vi "SDG60ConfArbWaveform3.vi"(0 "VISA resource name":refnum<visa-resource-name>="USB0::0xF4EC::0x1101::SDG6XEBC5R0119::INSTR", 1 "DDS/TArb 0: DDS":i32(ring) items=["DDS", "TrueArb"], 2 "Interpolation 0: Zero-order":i32(ring) items=["Zero-Order", "Linear", "Sinc", "Sin27", "Sinc13"], 3 "Offset (0.00 V)":dbl min=-10.0 max=10.0 format="%#_15g", 5 "Select Channel (1:Channel 1)":i32(ring)=1 items=["Channel 1"=1, "Channel 2"=2], 7 "Amplitude(0.1 Vpp)":dbl=0.1 min=0.001 max=20.0 step=1.0 format="%#.15f", 9 "Freq/SR/P (1 Hz)":dbl=1.0 min=1e-06 max=160000000.0 step=1.0 format="%#.15g", 11 "error in (no error)":errorcluster, 12 "Select Freq/SR/P (0:Freq)":i32(ring) items=["Frequency", "Sample Rate", "Period"], 13 "Phase (0 deg)":dbl min=-360.0 max=360.0 format="%#.15g") -> (4 "VISA resource name out":refnum<visa-resource-name>, 15 "error out":errorcluster)   [LabVIEW 2018]
doc: "Sets the waveform parameters for an arbitrary waveform. This VI should be called after <b>Create Arbitrary Waveform.vi</b> (for user defined arbitrary waveform) and <b>Select Arbitrary Waveform.vi</b>"
panel:
  # "Must precede with SDG60SelectArbitraryWFM\nMay take time (~20s) if WFM is large"
  # "Sinc type interpolations use virtual keys\nVirtual keys not used for zero-hold & linear\nInterpolation method, is only for TrueArb\nIf still selected, generator will not make any parameter changes"
  # "Range: 2mVpp-20Vpp. \n6 digits precision"
  # "Range: -10V-10V\n6 digits precision"
  # "Freq (DDS): 1uHz-50MHz \nFreq (TrueArb): 1uHz- Max depends on WFM length\nSR: 1uS/s-300MSa/s\nP: 20ns-1Ms\n10 Digit precision for F & SR\n6 Digit precision for P"
  # "May need more testing, as had issues\nwhere some of the parameters didn't go\nthrough the first time round"
  # "For TrueArb use only F or SR \nFor DDS use F or P\nMay take time (seconds to tens of secons!) to switch to TrueArb if WFM is large"
  # "Range -360..360deg, larger values will be warped to this range. Resolution 0.0001 deg"
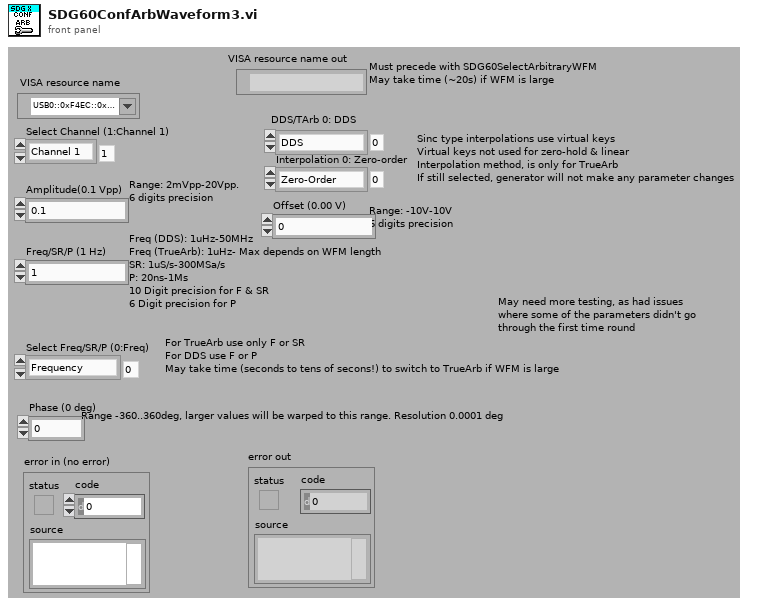
[diagram p1: front panel]
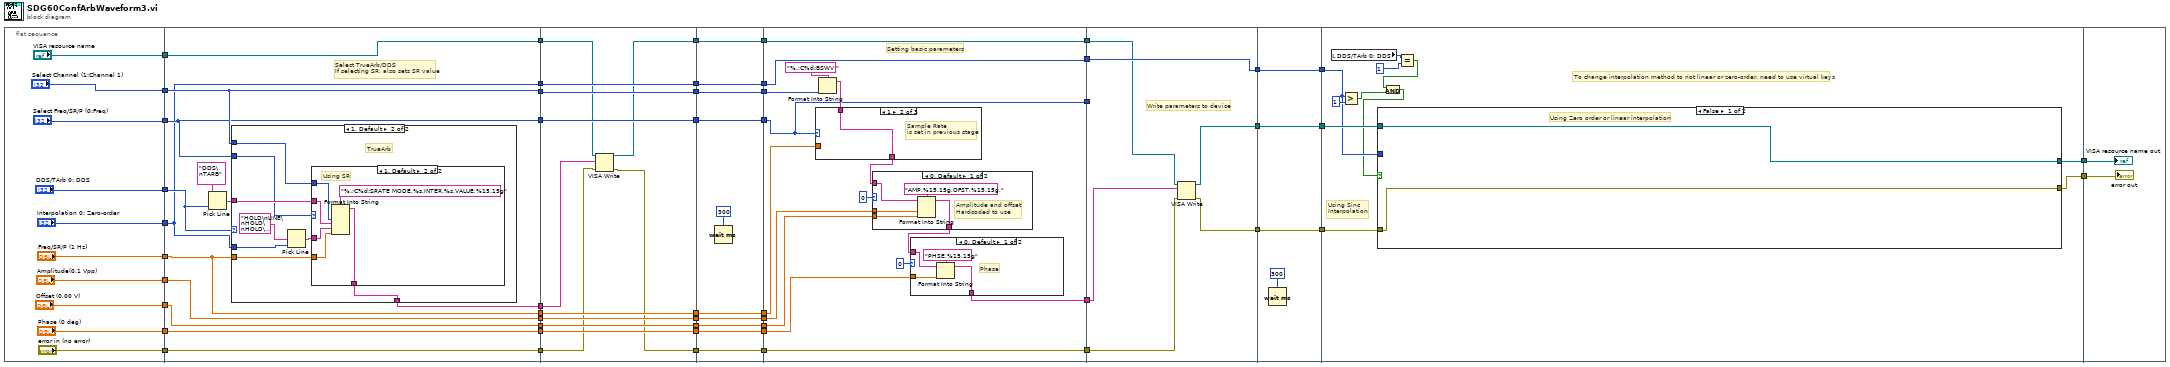
[diagram p0: block diagram]
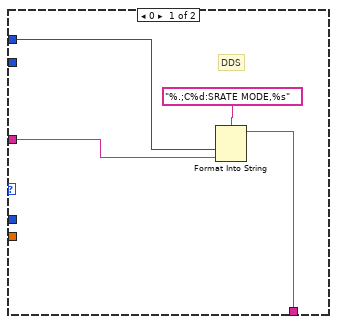
[diagram p2: hidden frame]
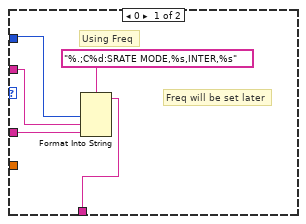
[diagram p3: hidden frame]
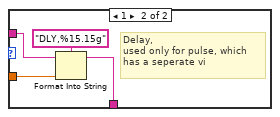
[diagram p4: hidden frame]
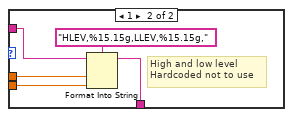
[diagram p5: hidden frame]
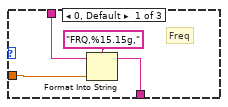
[diagram p6: hidden frame]
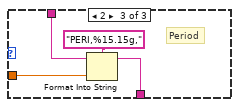
[diagram p7: hidden frame]
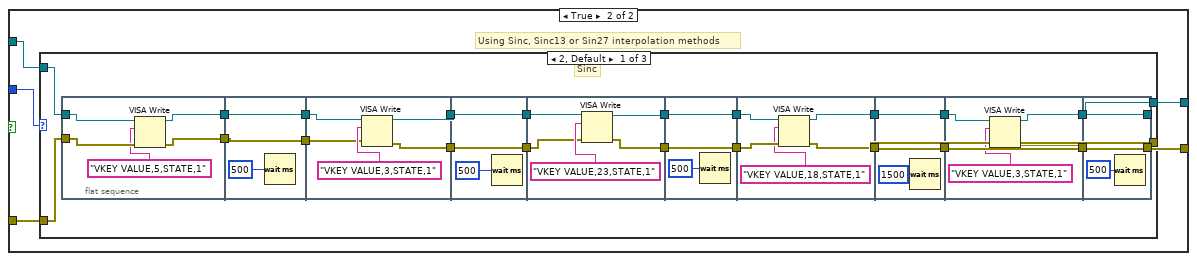
[diagram p8: hidden frame]
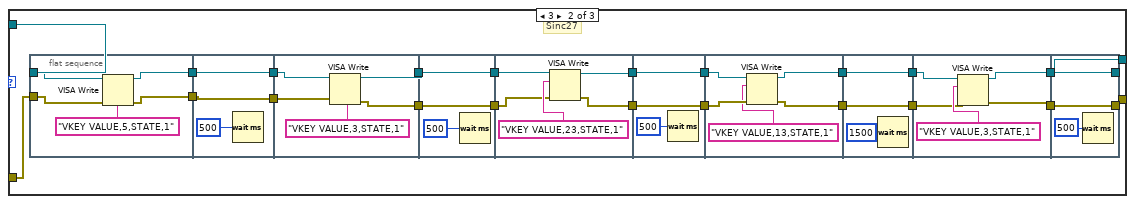
[diagram p9: hidden frame]
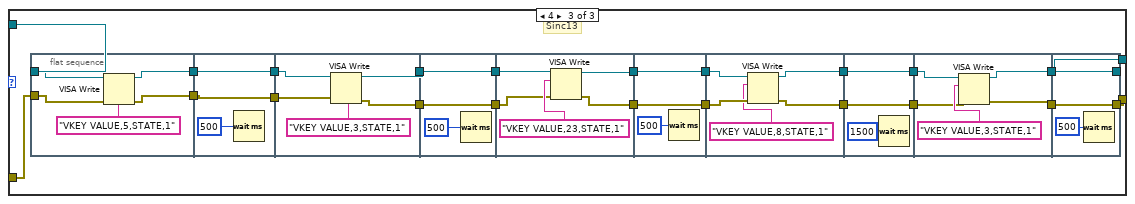
[diagram p10: hidden frame]
diagram:
  n1 = flat-sequence {
    tunnel: ["VISA resource name"] -> w51
    tunnel: ["error in (no error)"] -> w50
    tunnel: ["Amplitude(0.1 Vpp)"] -> w49
    tunnel: ["Phase (0 deg)"] -> w48
    tunnel: ["Freq/SR/P (1 Hz)"] -> w47
    tunnel: ["Offset (0.00 V)"] -> w46
    tunnel: ["Select Freq/SR/P (0:Freq)"] -> w45
    tunnel: ["DDS/TArb 0: DDS"] -> w44
    tunnel: ["Interpolation 0: Zero-order"] -> w43
    tunnel: ["Select Channel (1:Channel 1)"] -> w42
    tunnel: w51 -> [w70]
    tunnel: w50 -> [w74]
    tunnel: w49 -> [w68]
    tunnel: w48 -> [w69]
    tunnel: w47 -> [w67]
    tunnel: w46 -> [w66]
    tunnel: w45 -> [w64]
    tunnel: w44 -> [w71]
    tunnel: w43 -> [w63]
    tunnel: w42 -> [w65]
    tunnel: [w74] -> w34
    tunnel: [w70] -> w33
    tunnel: [w69] -> w32
    tunnel: [w68] -> w31
    tunnel: [w67] -> w30
    tunnel: [w66] -> w29
    tunnel: [w65] -> w28
    tunnel: [w64] -> w27
    tunnel: [w63] -> w26
    tunnel: [w62] -> w25
    tunnel: w34 -> [w100]
    tunnel: w33 -> [w102]
    tunnel: w32 -> [w109]
    tunnel: [w109] -> w22
    tunnel: w31 -> [w108]
    tunnel: [w108] -> w20
    tunnel: w30 -> [w107]
    tunnel: [w107] -> w18
    tunnel: w29 -> [w106]
    tunnel: [w106] -> w16
    tunnel: w28 -> [w105]
    tunnel: [w105] -> w14
    tunnel: w27 -> [w104]
    tunnel: [w104] -> w12
    tunnel: w26 -> [w103]
    tunnel: [w103] -> w10
    tunnel: w25 -> [w98]
    tunnel: [w101] -> w8
    tunnel: [w99] -> w7
    tunnel: [w119] -> w24
    tunnel: [w118] -> w23
    tunnel: w22 -> [w117]
    tunnel: [w117] -> w21
    tunnel: w20 -> [w116]
    tunnel: [w116] -> w19
    tunnel: w18 -> [w115]
    tunnel: [w115] -> w17
    tunnel: w16 -> [w114]
    tunnel: [w114] -> w15
    tunnel: w14 -> [w113]
    tunnel: [w113] -> w13
    tunnel: w12 -> [w112]
    tunnel: [w112] -> w11
    tunnel: w10 -> [w111]
    tunnel: [w111] -> w9
    tunnel: w8 -> [w118]
    tunnel: w7 -> [w119]
    tunnel: w24 -> [w135]
    tunnel: [w135] -> w41
    tunnel: w23 -> [w134]
    tunnel: [w134] -> w40
    tunnel: w21 -> [w125]
    tunnel: w19 -> [w127]
    tunnel: w17 -> [w128]
    tunnel: w15 -> [w126]
    tunnel: w13 -> [w129]
    tunnel: w11 -> [w120]
    tunnel: w9 -> [w124]
    tunnel: [w124] -> w39
    tunnel: [w123] -> w38
    tunnel: [w120] -> w35
    tunnel: w41 -> [w164]
    tunnel: w40 -> [w167]
    tunnel: w39 -> [w168]
    tunnel: w38 -> [w163]
    tunnel: [w166] -> w6
    tunnel: [w165] -> w4
    tunnel: [w168] -> w2
    tunnel: w35 -> [_]
    tunnel: w6 -> [w172]
    tunnel: [w172] -> w5
    tunnel: w4 -> [w171]
    tunnel: [w171] -> w3
    tunnel: w2 -> [w170]
    tunnel: [w170] -> w1
    tunnel: w5 -> [w181]
    tunnel: w3 -> [w182]
    tunnel: w1 -> [w178]
    tunnel: [w183] -> w37
    tunnel: [w180] -> w36
    tunnel: w37 -> [w378]
    tunnel: w36 -> [w377]
    frame #0 {
    }
    frame #1 {
      # "Select TrueArb/DDS\nIf selecting SR, also sets SR value"
      n2 = Pick Line(multi-line string="DDS\nTARB", line index=w71) -> (output string=w72:string)  [unwired: 1 in]
      n3 = case shown="1, Default" w71 {
        tunnel: [w77 w86] -> w62
        tunnel: w65 -> [w75 w85]
        tunnel: w72 -> [w76 w84]
        tunnel: w67 -> [_ w81]
        tunnel: w64 -> [_ w80]
        tunnel: w63 -> [_ w79]
        frame 0 {
          # "DDS"
          n4 = Format Into String(format string="%.;C%d:SRATE MODE,%s", w75, w76) -> (resulting string=w77:string)  [unwired: 2 in, 1 out]
        }
        frame 1, Default {
          # "TrueArb"
          n5 = Pick Line(multi-line string="HOLD\nLINE\nHOLD\nHOLD\nHOLD\nHOLD", line index=w79) -> (output string=w82:string)  [unwired: 1 in]
          n6 = case shown="1, Default" w80 {
            tunnel: w85 -> [w90 w96]
            tunnel: [w89 w95] -> w86
            tunnel: w84 -> [w88 w94]
            tunnel: w82 -> [w87 w93]
            tunnel: w81 -> [_ w92]
            frame 0 {
              # "Freq will be set later"
              # "Using Freq"
              n7 = Format Into String(format string="%.;C%d:SRATE MODE,%s,INTER,%s", w90, w88, w87) -> (resulting string=w89:string)  [unwired: 2 in, 1 out]
            }
            frame 1, Default {
              # "Using SR"
              n8 = Format Into String(format string="%.;C%d:SRATE MODE,%s,INTER,%s,VALUE,%15.15g", w96, w94, w93, w92) -> (resulting string=w95:string)  [unwired: 2 in, 1 out]
            }
          }
        }
      }
    }
    frame #2 {
      n9 = VISA Write(VISA resource name=w102, write buffer=w98, error in (no error)=w100) -> (VISA resource name out=w101:refnum<visa-resource-name>, error out=w99:errorcluster)  [unwired: 1 out]
    }
    frame #3 {
      n10 = Wait (ms)(milliseconds to wait=300 ("x")) -> ()  [unwired: 1 out]
    }
    frame #4 {
      # "Setting basic parameters"
      n11 = Format Into String(format string="%.;C%d:BSWV ", w129) -> (resulting string=w131:string)  [unwired: 2 in, 1 out]
      n12 = case shown="1" w120 {
        tunnel: w131 -> [w157 w158 w162]
        tunnel: [w155 w158 w160] -> w121
        tunnel: w128 -> [w154 _ w159]
        frame 0, Default {
          # "Freq"
          n13 = Format Into String(format string="FRQ,%15.15g,", initial string=w157, w154) -> (resulting string=w155:string)  [unwired: 1 in, 1 out]
        }
        frame 1 {
          # "Sample Rate\nis set in previous stage"
        }
        frame 2 {
          # "Period"
          n14 = Format Into String(format string="PERI,%15.15g,", initial string=w162, w159) -> (resulting string=w160:string)  [unwired: 1 in, 1 out]
        }
      }
      n15 = case shown="0, Default" 0 {
        tunnel: [w147 w152] -> w122
        tunnel: w127 -> [w146 w151]
        tunnel: w126 -> [w145 w150]
        tunnel: w121 -> [w144 w149]
        frame 0, Default {
          # "Amplitude and offset\nHardcoded to use"
          n16 = Format Into String(format string="AMP,%15.15g,OFST,%15.15g,", initial string=w144, w146, w145) -> (resulting string=w147:string)  [unwired: 1 in, 1 out]
        }
        frame 1 {
          # "High and low level\nHardcoded not to use"
          n17 = Format Into String(format string="HLEV,%15.15g,LLEV,%15.15g,", initial string=w149, w151, w150) -> (resulting string=w152:string)  [unwired: 1 in, 1 out]
        }
      }
      n18 = case shown="0, Default" 0 {
        tunnel: [w138 w142] -> w123
        tunnel: w125 -> [w137 w141]
        tunnel: w122 -> [w136 w140]
        frame 0, Default {
          # "Phase"
          n19 = Format Into String(format string="PHSE,%15.15g", initial string=w136, w137) -> (resulting string=w138:string)  [unwired: 1 in, 1 out]
        }
        frame 1 {
          # "Delay,\nused only for pulse, which \nhas a seperate vi"
          n20 = Format Into String(format string="DLY,%15.15g", initial string=w140, w141) -> (resulting string=w142:string)  [unwired: 1 in, 1 out]
        }
      }
    }
    frame #5 {
      # "Write parameters to device"
      n21 = VISA Write(VISA resource name=w167, write buffer=w163, error in (no error)=w164) -> (VISA resource name out=w165:refnum<visa-resource-name>, error out=w166:errorcluster)  [unwired: 1 out]
    }
    frame #6 {
      n22 = Wait (ms)(milliseconds to wait=300 ("x")) -> ()  [unwired: 1 out]
    }
    frame #7 {
      # "Using Sinc \nInterpolation"
      # "To change interpolation method to not linear or zero-order, need to use virtual keys"
      n23 = local read "DDS/TArb 0: DDS"() -> (w177:i32)
      n24 = Greater?(x=w178, y=1) -> (0:w174:bool)
      n25 = Equal?(x=w177, y=1) -> (x = y?=w175:bool)
      n26 = And(x=w175, y=w174) -> (x .and. y?=w173:bool)
      n27 = case shown="False" w173 {
        tunnel: [w185 w187] -> w183
        tunnel: [w184 w188] -> w180
        tunnel: w182 -> [w185 w190]
        tunnel: w181 -> [w184 w189]
        tunnel: w178 -> [_ w186]
        frame False {
          # "Using Zero order or linear interpolation"
        }
        frame True {
          # "Using Sinc, Sinc13 or Sin27 interpolation methods"
          n28 = case shown="2, Default" w186 {
            tunnel: w190 -> [w207 w269 w331]
            tunnel: w189 -> [w208 w270 w332]
            tunnel: [w205 w267 w329] -> w188
            tunnel: [w206 w268 w330] -> w187
            frame 2, Default {
              # "Sinc"
              n29 = flat-sequence {
                tunnel: w208 -> [w217]
                tunnel: w207 -> [w216]
                tunnel: [w215] -> w212
                tunnel: [w213] -> w211
                tunnel: w212 -> [w220]
                tunnel: [w220] -> w210
                tunnel: [w218] -> w209
                tunnel: w211 -> [w218]
                tunnel: w210 -> [w224]
                tunnel: w209 -> [w221]
                tunnel: [w223] -> w204
                tunnel: [w222] -> w203
                tunnel: w204 -> [w228]
                tunnel: [w228] -> w202
                tunnel: w203 -> [w227]
                tunnel: [w227] -> w200
                tunnel: w202 -> [w233]
                tunnel: [w229] -> w201
                tunnel: w200 -> [w231]
                tunnel: [w230] -> w199
                tunnel: w201 -> [w236]
                tunnel: w199 -> [w235]
                tunnel: [w236] -> w198
                tunnel: [w235] -> w197
                tunnel: w198 -> [w241]
                tunnel: w197 -> [w240]
                tunnel: [w238] -> w196
                tunnel: [w239] -> w195
                tunnel: w196 -> [w244]
                tunnel: w195 -> [w243]
                tunnel: [w244] -> w194
                tunnel: [w243] -> w193
                tunnel: w194 -> [w249]
                tunnel: w193 -> [w246]
                tunnel: [w248] -> w192
                tunnel: [w245] -> w191
                tunnel: [w251] -> w205
                tunnel: [w252] -> w206
                tunnel: w192 -> [w252]
                tunnel: w191 -> [w251]
                frame #0 {
                  n30 = VISA Write(VISA resource name=w216, write buffer="VKEY VALUE,5,STATE,1", error in (no error)=w217) -> (VISA resource name out=w215:refnum<visa-resource-name>, error out=w213:errorcluster)  [unwired: 1 out]
                }
                frame #1 {
                  n31 = Wait (ms)(milliseconds to wait=500) -> ()  [unwired: 1 out]
                }
                frame #2 {
                  n32 = VISA Write(VISA resource name=w224, write buffer="VKEY VALUE,3,STATE,1", error in (no error)=w221) -> (VISA resource name out=w223:refnum<visa-resource-name>, error out=w222:errorcluster)  [unwired: 1 out]
                }
                frame #3 {
                  n33 = Wait (ms)(milliseconds to wait=500) -> ()  [unwired: 1 out]
                }
                frame #4 {
                  n34 = VISA Write(VISA resource name=w233, write buffer="VKEY VALUE,23,STATE,1", error in (no error)=w231) -> (VISA resource name out=w229:refnum<visa-resource-name>, error out=w230:errorcluster)  [unwired: 1 out]
                }
                frame #5 {
                  n35 = Wait (ms)(milliseconds to wait=500) -> ()  [unwired: 1 out]
                }
                frame #6 {
                  n36 = VISA Write(VISA resource name=w241, write buffer="VKEY VALUE,18,STATE,1", error in (no error)=w240) -> (VISA resource name out=w238:refnum<visa-resource-name>, error out=w239:errorcluster)  [unwired: 1 out]
                }
                frame #7 {
                  n37 = Wait (ms)(milliseconds to wait=1500) -> ()  [unwired: 1 out]
                }
                frame #8 {
                  n38 = VISA Write(VISA resource name=w249, write buffer="VKEY VALUE,3,STATE,1", error in (no error)=w246) -> (VISA resource name out=w248:refnum<visa-resource-name>, error out=w245:errorcluster)  [unwired: 1 out]
                }
                frame #9 {
                  n39 = Wait (ms)(milliseconds to wait=500) -> ()  [unwired: 1 out]
                }
              }
            }
            frame 3 {
              # "Sinc27"
              n40 = flat-sequence {
                tunnel: w270 -> [w279]
                tunnel: w269 -> [w278]
                tunnel: [w277] -> w274
                tunnel: [w275] -> w273
                tunnel: w274 -> [w282]
                tunnel: [w282] -> w272
                tunnel: [w280] -> w271
                tunnel: w273 -> [w280]
                tunnel: w272 -> [w286]
                tunnel: w271 -> [w283]
                tunnel: [w285] -> w266
                tunnel: [w284] -> w265
                tunnel: w266 -> [w290]
                tunnel: [w290] -> w264
                tunnel: w265 -> [w289]
                tunnel: [w289] -> w262
                tunnel: w264 -> [w295]
                tunnel: [w291] -> w263
                tunnel: w262 -> [w293]
                tunnel: [w292] -> w261
                tunnel: w263 -> [w298]
                tunnel: w261 -> [w297]
                tunnel: [w298] -> w260
                tunnel: [w297] -> w259
                tunnel: w260 -> [w303]
                tunnel: w259 -> [w302]
                tunnel: [w300] -> w258
                tunnel: [w301] -> w257
                tunnel: w258 -> [w306]
                tunnel: w257 -> [w305]
                tunnel: [w306] -> w256
                tunnel: [w305] -> w255
                tunnel: w256 -> [w311]
                tunnel: w255 -> [w308]
                tunnel: [w310] -> w254
                tunnel: [w307] -> w253
                tunnel: [w313] -> w267
                tunnel: [w314] -> w268
                tunnel: w254 -> [w314]
                tunnel: w253 -> [w313]
                frame #0 {
                  n41 = VISA Write(VISA resource name=w278, write buffer="VKEY VALUE,5,STATE,1", error in (no error)=w279) -> (VISA resource name out=w277:refnum<visa-resource-name>, error out=w275:errorcluster)  [unwired: 1 out]
                }
                frame #1 {
                  n42 = Wait (ms)(milliseconds to wait=500) -> ()  [unwired: 1 out]
                }
                frame #2 {
                  n43 = VISA Write(VISA resource name=w286, write buffer="VKEY VALUE,3,STATE,1", error in (no error)=w283) -> (VISA resource name out=w285:refnum<visa-resource-name>, error out=w284:errorcluster)  [unwired: 1 out]
                }
                frame #3 {
                  n44 = Wait (ms)(milliseconds to wait=500) -> ()  [unwired: 1 out]
                }
                frame #4 {
                  n45 = VISA Write(VISA resource name=w295, write buffer="VKEY VALUE,23,STATE,1", error in (no error)=w293) -> (VISA resource name out=w291:refnum<visa-resource-name>, error out=w292:errorcluster)  [unwired: 1 out]
                }
                frame #5 {
                  n46 = Wait (ms)(milliseconds to wait=500) -> ()  [unwired: 1 out]
                }
                frame #6 {
                  n47 = VISA Write(VISA resource name=w303, write buffer="VKEY VALUE,13,STATE,1", error in (no error)=w302) -> (VISA resource name out=w300:refnum<visa-resource-name>, error out=w301:errorcluster)  [unwired: 1 out]
                }
                frame #7 {
                  n48 = Wait (ms)(milliseconds to wait=1500) -> ()  [unwired: 1 out]
                }
                frame #8 {
                  n49 = VISA Write(VISA resource name=w311, write buffer="VKEY VALUE,3,STATE,1", error in (no error)=w308) -> (VISA resource name out=w310:refnum<visa-resource-name>, error out=w307:errorcluster)  [unwired: 1 out]
                }
                frame #9 {
                  n50 = Wait (ms)(milliseconds to wait=500) -> ()  [unwired: 1 out]
                }
              }
            }
            frame 4 {
              # "Sinc13"
              n51 = flat-sequence {
                tunnel: w332 -> [w341]
                tunnel: w331 -> [w340]
                tunnel: [w339] -> w336
                tunnel: [w337] -> w335
                tunnel: w336 -> [w344]
                tunnel: [w344] -> w334
                tunnel: [w342] -> w333
                tunnel: w335 -> [w342]
                tunnel: w334 -> [w348]
                tunnel: w333 -> [w345]
                tunnel: [w347] -> w328
                tunnel: [w346] -> w327
                tunnel: w328 -> [w352]
                tunnel: [w352] -> w326
                tunnel: w327 -> [w351]
                tunnel: [w351] -> w324
                tunnel: w326 -> [w357]
                tunnel: [w353] -> w325
                tunnel: w324 -> [w355]
                tunnel: [w354] -> w323
                tunnel: w325 -> [w360]
                tunnel: w323 -> [w359]
                tunnel: [w360] -> w322
                tunnel: [w359] -> w321
                tunnel: w322 -> [w365]
                tunnel: w321 -> [w364]
                tunnel: [w362] -> w320
                tunnel: [w363] -> w319
                tunnel: w320 -> [w368]
                tunnel: w319 -> [w367]
                tunnel: [w368] -> w318
                tunnel: [w367] -> w317
                tunnel: w318 -> [w373]
                tunnel: w317 -> [w370]
                tunnel: [w372] -> w316
                tunnel: [w369] -> w315
                tunnel: [w375] -> w329
                tunnel: [w376] -> w330
                tunnel: w316 -> [w376]
                tunnel: w315 -> [w375]
                frame #0 {
                  n52 = VISA Write(VISA resource name=w340, write buffer="VKEY VALUE,5,STATE,1", error in (no error)=w341) -> (VISA resource name out=w339:refnum<visa-resource-name>, error out=w337:errorcluster)  [unwired: 1 out]
                }
                frame #1 {
                  n53 = Wait (ms)(milliseconds to wait=500) -> ()  [unwired: 1 out]
                }
                frame #2 {
                  n54 = VISA Write(VISA resource name=w348, write buffer="VKEY VALUE,3,STATE,1", error in (no error)=w345) -> (VISA resource name out=w347:refnum<visa-resource-name>, error out=w346:errorcluster)  [unwired: 1 out]
                }
                frame #3 {
                  n55 = Wait (ms)(milliseconds to wait=500) -> ()  [unwired: 1 out]
                }
                frame #4 {
                  n56 = VISA Write(VISA resource name=w357, write buffer="VKEY VALUE,23,STATE,1", error in (no error)=w355) -> (VISA resource name out=w353:refnum<visa-resource-name>, error out=w354:errorcluster)  [unwired: 1 out]
                }
                frame #5 {
                  n57 = Wait (ms)(milliseconds to wait=500) -> ()  [unwired: 1 out]
                }
                frame #6 {
                  n58 = VISA Write(VISA resource name=w365, write buffer="VKEY VALUE,8,STATE,1", error in (no error)=w364) -> (VISA resource name out=w362:refnum<visa-resource-name>, error out=w363:errorcluster)  [unwired: 1 out]
                }
                frame #7 {
                  n59 = Wait (ms)(milliseconds to wait=1500) -> ()  [unwired: 1 out]
                }
                frame #8 {
                  n60 = VISA Write(VISA resource name=w373, write buffer="VKEY VALUE,3,STATE,1", error in (no error)=w370) -> (VISA resource name out=w372:refnum<visa-resource-name>, error out=w369:errorcluster)  [unwired: 1 out]
                }
                frame #9 {
                  n61 = Wait (ms)(milliseconds to wait=500) -> ()  [unwired: 1 out]
                }
              }
            }
          }
        }
      }
    }
    frame #8 {
      "VISA resource name out" <- w378
      "error out" <- w377
    }
  }
